vi "TCP Read - Terminated String.vi"(7 "Termination Character":string="\n", 8 "error in":errorcluster, 9 "Timeout ms (default 50ms)":i32=50, 11 "TCP Network Connection in":refnum<k5>) -> (0 "error out":errorcluster, 2 "Read String":string, 3 "TCP Network Connection out":refnum<k5>)   [LabVIEW 2017, in "Communications Library.lvlib"]
doc: "Reads characters one by one from the TCP port.\n\nExits, when the termination character is received or the timeout expires."
uses:
  Communications Library.lvlib
  Error 5102 - DTACQ unit replied with an error--const.vi
  Debug - TCP - Write to Log File.vi
  Debug - TCP - Create Descriptive String.vi
  <vilib>/Utility/error.llb/Error Cluster From Error Code.vi
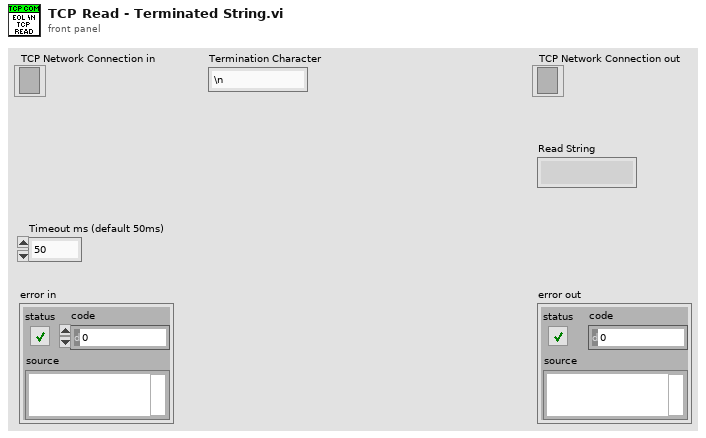
[diagram p1: front panel]
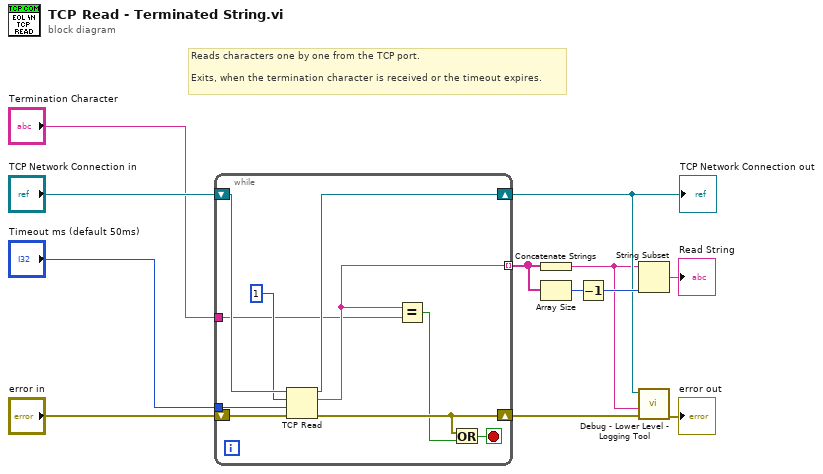
[diagram p0: block diagram]
diagram:
  # "Reads characters one by one from the TCP port.\n\nExits, when the termination character is received or the timeout expires."
  n1 = while {
    tunnel: [w16] -> w9 mode=indexing
    shift-right: [w17] -> w4
    shift-left: "error in" -> [w21]
    shift-right: [w22] -> w2
    shift-left: "TCP Network Connection in" -> [w20]
    tunnel: "Timeout ms (default 50ms)" -> [w18]
    tunnel: "Termination Character" -> [w13]
    stop <- w14 stop-if-true
    n2 = TCP Read(connection ID=w20, bytes to read=1, error in (no error)=w21, 9:w18) -> (connection ID out=w22:refnum<k5>, data out=w16:string, error out=w17:errorcluster)  [unwired: 1 in]
    n3 = Equal?(x=w16, y=w13) -> (x = y?=w15:bool)
    n4 = Or(x=w17, y=w15) -> (x .or. y?=w14:bool)
  }
  "TCP Network Connection out" <- w2
  n5 = Concatenate Strings(w9) -> (w1:string)
  n6 = Array Size(array=w9) -> (size(s)=w8:i32)
  n7 = Decrement(x=w8) -> (x-1=w7:i32)
  n8 = String Subset(string=w1, length (rest)=w7) -> (substring=→"Read String":string)  [unwired: 1 in]
  n9 = call "Debug - Lower Level - Logging Tool.vi"("Error In"=w4, "Data Received"=w1, "TCP Network Connecion In"=w2) -> ("Error Out"=→"error out":errorcluster)  [unwired: 7 in, 1 out]
